vi "Write Base Path For Task Files.vi"(8 "error in (no error)":errorcluster, 10 "Base Path For Task Files":path=path "c:/IntanTasks", 11 "IntanElectrophysiology in":refnum<class "IntanElectrophysiology.lvclass">) -> (0 "error out":errorcluster, 3 "IntanElectrophysiology out":refnum<class "IntanElectrophysiology.lvclass">)   [LabVIEW 2014, in "IntanElectrophysiology.lvclass"]
uses:
  IntanElectrophysiology.lvclass
  IntanElectrophysiology.lvclass/IntanElectrophysiology.ctl
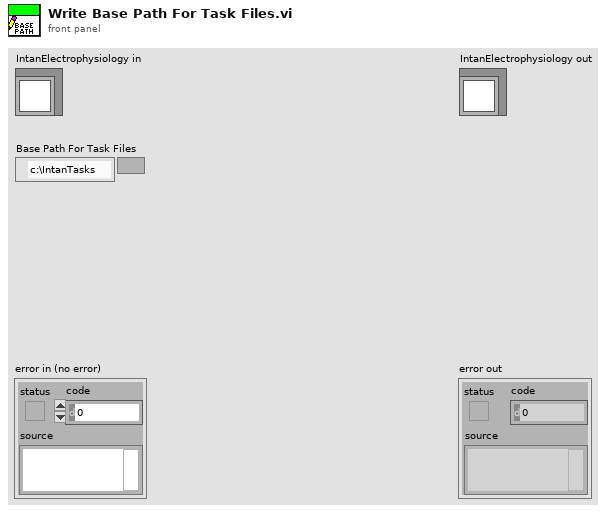
[diagram p1: front panel]
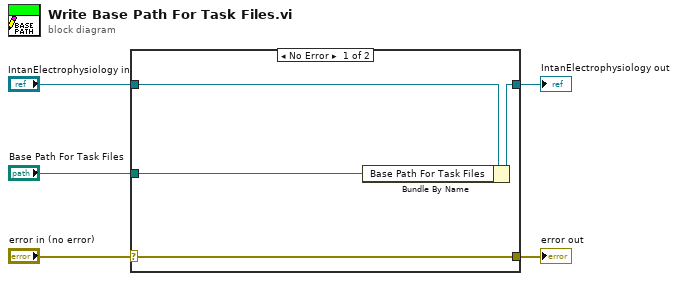
[diagram p0: block diagram]
diagram:
  n1 = case shown="No Error" "error in (no error)" {
    selector: "error in (no error)" -> [w9 w10]
    tunnel: [w9 w10] -> w4
    tunnel: [w7 w11] -> w2
    tunnel: "IntanElectrophysiology in" -> [w8 w11]
    tunnel: "Base Path For Task Files" -> [w6 _]
    frame No Error {
      n2 = Bundle By Name(cluster=w8, "Base Path For Task Files"=w6) -> (w7:refnum<class "IntanElectrophysiology.lvclass">)
    }
    frame Error {
    }
  }
  "error out" <- w4
  "IntanElectrophysiology out" <- w2
